vi "Fetch Base Class Info.vi"(8 "error in (no error)":errorcluster, 11 "LVClassLibrary in":refnum<vi>) -> (0 "error out":errorcluster, 2 "Base Class Info":T1, 3 "LVClassLibrary out":refnum<vi>)   [LabVIEW 2023, in "VIDoc Parsing.lvlib"]
uses:
  VIDoc Parsing.lvlib
  TypeDefs/Base Class Info Cluster.ctl
  <vilib>/picture/picture.llb/imagedata.ctl
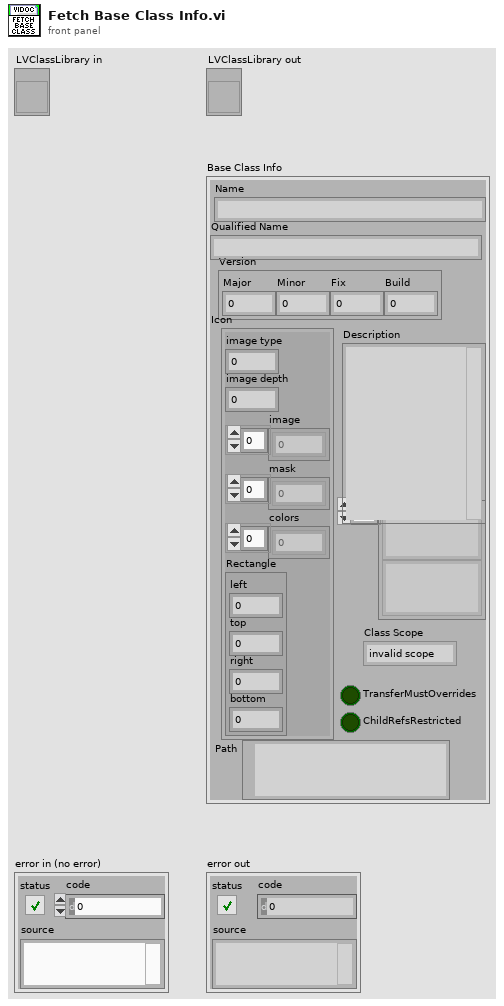
[diagram p1: front panel]
types:
  T1 = typedef "VIDoc Parsing.lvlib/Base Class Info Cluster.ctl" = cluster{"Name":string, "Icon":T2, "Version":cluster{"Major":u16, "Minor":u16, "Fix":u16, "Build":u16}, "Description":string, "Friends":string[], "ChildRefsRestricted":bool, "TransferMustOverrides":bool, "Path":path, "Qualified Name":string, "Class Scope":enum32{"invalid scope", "public", "private", "protected", "community"}}
  T2 = typedef "imagedata.ctl" = cluster{"image type":i32, "image depth":i32, "image":u8[], "mask":u8[], "colors":u32[], "Rectangle":cluster{"left":i16, "top":i16, "right":i16, "bottom":i16}}
  T3 = enum32{"invalid scope", "public", "private", "protected", "community"}
  T4 = cluster{"Major":u16, "Minor":u16, "Fix":u16, "Build":u16}
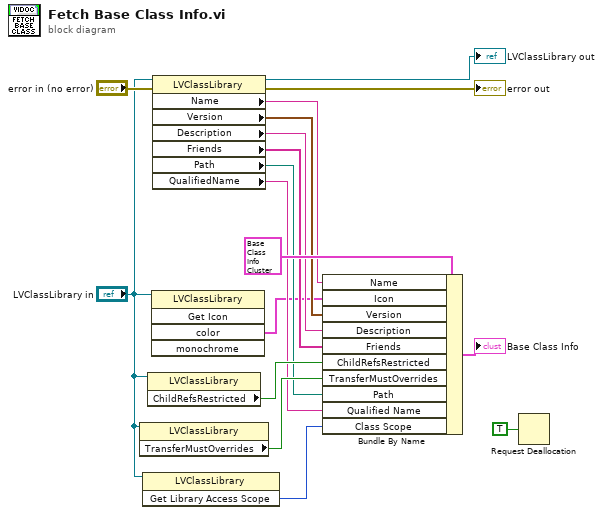
[diagram p0: block diagram]
diagram:
  n1 = property class="LVClassLibrary"(reference="LVClassLibrary in") -> ("TransferMustOverrides"=w7:bool)  [unwired: 1 in, 2 out]
  n2 = invoke class="LVClassLibrary" method="Get Library Access Scope"(reference="LVClassLibrary in") -> ("Get Library Access Scope"=w1:T3)  [unwired: 2 in, 2 out]
  n3 = property class="LVClassLibrary"(reference="LVClassLibrary in") -> ("ChildRefsRestricted"=w8:bool)  [unwired: 1 in, 2 out]
  n4 = invoke class="LVClassLibrary" method="Get Icon"(reference="LVClassLibrary in") -> ("color"=w3:T2)  [unwired: 4 in, 4 out]
  n5 = property class="LVClassLibrary"(reference="LVClassLibrary in", error in="error in (no error)") -> (reference out=→"LVClassLibrary out":refnum<vi>, error out=→"error out":errorcluster, "Name"=w10:string, "Version"=w11:T4, "Description"=w12:string, "Friends"=w14:string[], "Path"=w5:path, "QualifiedName"=w4:string)
  n6 = Bundle By Name(cluster=T1 {"Name"="", "Icon"={"image type"=0, "image depth"=0, "image"=[], "mask"=[], "colors"=[], "Rectangle"={"left"=0, "top"=0, "right"=0, "bottom"=0}}, "Version"={"Major"=0, "Minor"=0, "Fix"=0, "Build"=0}, "Description"="", "Friends"=[], "ChildRefsRestricted"=FALSE, "TransferMustOverrides"=FALSE, "Path"=path "", "Qualified Name"="", "Class Scope"=enum."invalid scope"} ("cluster in"), "Name"=w10, "Icon"=w3, "Version"=w11, "Description"=w12, "Friends"=w14, "ChildRefsRestricted"=w8, "TransferMustOverrides"=w7, "Path"=w5, "Qualified Name"=w4, "Class Scope"=w1) -> (→"Base Class Info":T1)
  n7 = Request Deallocation(TRUE ("flag")) -> ()
